vi "Initialize.vi"(8 "error in (no error)":errorcluster, 11 "[P] User in":refnum<class "[P] User.lvclass">) -> (0 "error out":errorcluster, 3 "[P] User out":refnum<class "[P] User.lvclass">)   [LabVIEW 2020, in "[P] User.lvlib" / "[P] User.lvclass"]
uses:
  [P] User.lvclass
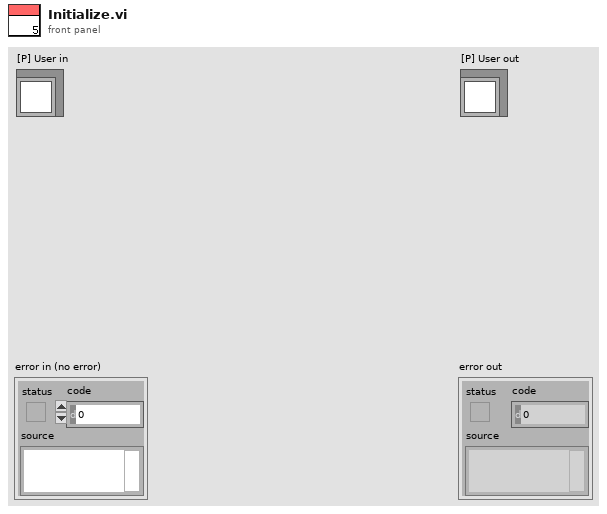
[diagram p1: front panel]
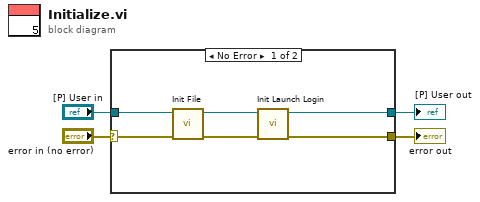
[diagram p0: block diagram]
diagram:
  n1 = case shown="No Error" "error in (no error)" {
    selector: "error in (no error)" -> [w10 w12]
    tunnel: [w5 w12] -> w3
    tunnel: [w6 w11] -> w1
    tunnel: "[P] User in" -> [w9 w11]
    frame No Error {
      n2 = call "Init File.vi"("error in (no error)"=w10, "[P] User in"=w9) -> ("error out"=w7:errorcluster, "[P] User out"=w8:refnum<class "[P] User.lvclass">)  [unwired: 8 in]
      n3 = call "Init Launch Login.vi"("error in (no error)"=w7, "[P] User in"=w8) -> ("error out"=w5:errorcluster, "[P] User out"=w6:refnum<class "[P] User.lvclass">)  [unwired: 8 in]
    }
    frame Error {
    }
  }
  "error out" <- w3
  "[P] User out" <- w1
